vi "AdjustFlyback.vi"(8 "error in (no error)":errorcluster, 11 "Microscope in":refnum<class "Microscope.lvclass">) -> (0 "error out":errorcluster, 3 "Microscope out":refnum<class "Microscope.lvclass">)   [LabVIEW 2012, in "Microscope.lvclass"]
uses:
  classes/Microscope.lvclass
  classes/Microscope.lvclass/Microscope.ctl
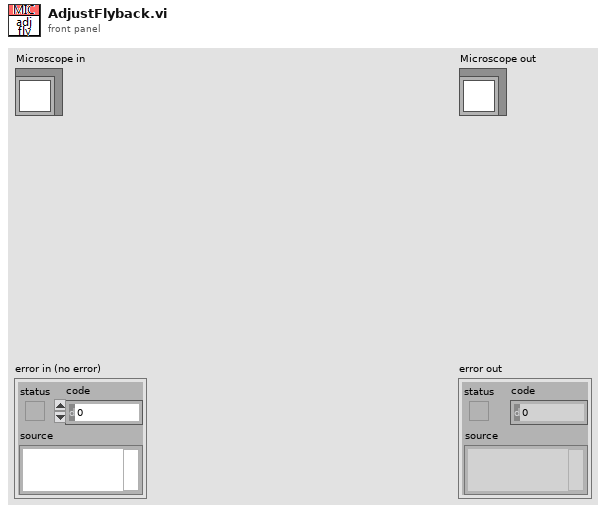
[diagram p1: front panel]
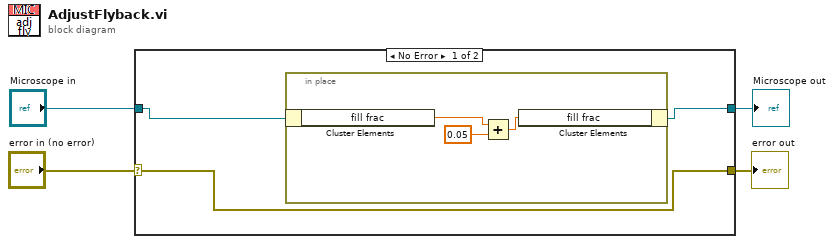
[diagram p0: block diagram]
diagram:
  n1 = case shown="No Error" "error in (no error)" {
    selector: "error in (no error)" -> [w5 w12]
    tunnel: [w5 w12] -> w3
    tunnel: [w6 w11] -> w1
    tunnel: "Microscope in" -> [w7 w11]
    frame No Error {
      n2 = in-place {
        n3 = in-place-cluster #1(w7) -> ("fill frac"=w9:dbl)
        n4 = Add(x=w9, y=0.05) -> (x+y=w8:dbl)
        n5 = in-place-cluster #1("fill frac"=w8) -> (w6:refnum<class "Microscope.lvclass">)
      }
    }
    frame Error {
    }
  }
  "error out" <- w3
  "Microscope out" <- w1
